vi "MiseEnFormeStreamMesuresValise.vi"(4 "Error In":errorcluster caption="Entrée d'erreur", 6 "MesuresBrutesValise":dbl[](array[numeric])=[1.0, 1.0, 1.0, 1.0, 1.0, 1.0, 1.0, 1.0, 1.0, 1.0, 1.0, 1.0, 1.0, 1.0, 1.0, 1.0, 1.0, 1.0, 1.0, 1.0, 1.0, 1.0, 1.0, 1.0], 7 "ConfigTotale":T1={"VoltageChannels"={"ChannelNames"=["capteur1", "capteur2"], "Sensitivity(Unit/V)"=[1.0, 1.0], "AutoZero"=[FALSE, FALSE], "ChannelUnits"=["V", "V"], "Offsets(Units)"=[0.0, 0.0], "Graph Num"=[]}, "WheastoneBridgeChannels"={"ChannelNames"=["capteur1", "capteur2"], "Sensitivity(Unit/V)"=[1.0, 1.0], "AutoZero"=[FALSE, FALSE], "ChannelUnits"=["V", "V"], "Offsets(Units)"=[0.0, 0.0], "Graph Num"=[]}, "Configuration"={"AcqSamplingRate(Hz)"=1000, "AcqTime(s)"=10, "Trigger"=FALSE, "NbVoltageChannels"=2, "NbWBridgeChannels"=2, "Qualisys"=FALSE, "Hexapode"=FALSE, "FinalSamplingRate(Hz)"=100, "QualisysDataType"=enum."6DOF", "Nortek"=FALSE, "HBM"=FALSE}}) -> (0 "Error Out":errorcluster caption="Sortie d'erreur", 2 "VoltageChannels1(0to15)":dbl[](array[numeric])=[1.0, 1.0], 3 "WBridgeChannels":dbl[](array[numeric])=[1000.0, 1000.0])   [LabVIEW 2017]
uses:
  DefDeType/ConfigTotale.ctl
  DefDeType/VoltageChannels.ctl
  DefDeType/WBridgeChannels.ctl
  DefDeType/Configuration.ctl
panel:
  out "size(s)":i32
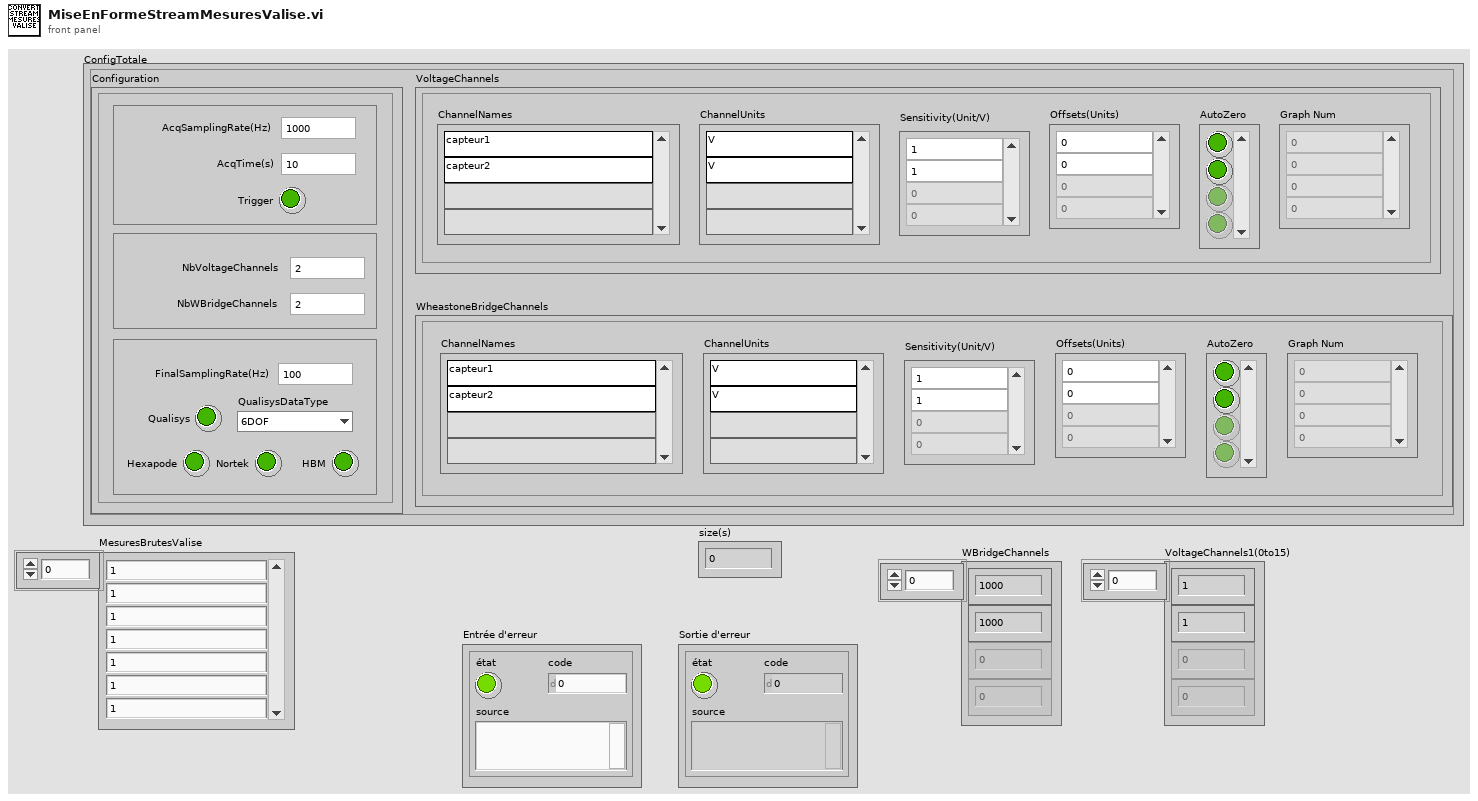
[diagram p1: front panel]
types:
  T1 = typedef "ConfigTotale.ctl" = cluster{"VoltageChannels":T2, "WheastoneBridgeChannels":T3, "Configuration":T4}
  T2 = typedef "VoltageChannels.ctl" = cluster{"ChannelNames":string[], "Sensitivity(Unit/V)":dbl[], "AutoZero":bool[], "ChannelUnits":string[], "Offsets(Units)":dbl[], "Graph Num":u8[]}
  T3 = typedef "WBridgeChannels.ctl" = cluster{"ChannelNames":string[], "Sensitivity(Unit/V)":dbl[], "AutoZero":bool[], "ChannelUnits":string[], "Offsets(Units)":dbl[], "Graph Num":u8[]}
  T4 = typedef "Configuration.ctl" = cluster{"AcqSamplingRate(Hz)":u32, "AcqTime(s)":u32, "Trigger":bool, "NbVoltageChannels":u32, "NbWBridgeChannels":u32, "Qualisys":bool, "Hexapode":bool, "FinalSamplingRate(Hz)":u32, "QualisysDataType":enum16{"6DOF", "3DTracking", "6DOF + 3D"}, "Nortek":bool, "HBM":bool}
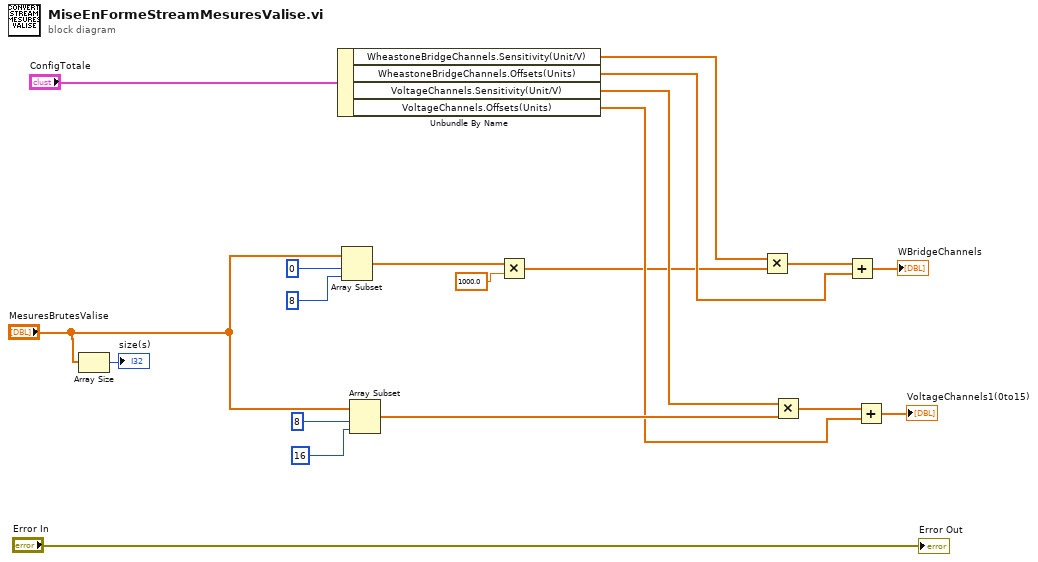
[diagram p0: block diagram]
diagram:
  n1 = Array Size(array="MesuresBrutesValise") -> (size(s)=→"size(s)":i32)
  n2 = Unbundle By Name("ConfigTotale") -> ("WheastoneBridgeChannels.Sensitivity(Unit/V)"=w13:dbl[], "WheastoneBridgeChannels.Offsets(Units)"=w12:dbl[], "VoltageChannels.Sensitivity(Unit/V)"=w15:dbl[], "VoltageChannels.Offsets(Units)"=w11:dbl[])
  n3 = Array Subset(array="MesuresBrutesValise", index=0 ("indice"), length=8 ("longueur")) -> (w4:dbl[])
  n4 = Array Subset(array="MesuresBrutesValise", index=8 ("indice"), length=16 ("longueur")) -> (w16:dbl[])
  n5 = Multiply(x=w4, y=1000.0) -> (x*y=w5:dbl[])
  n6 = Multiply(x=w13, y=w5) -> (x*y=w14:dbl[])
  n7 = Multiply(x=w15, y=w16) -> (x*y=w10:dbl[])
  n8 = Add(x=w14, y=w12) -> (x+y=→"WBridgeChannels":dbl[])
  n9 = Add(x=w10, y=w11) -> (x+y=→"VoltageChannels1(0to15)":dbl[])
  "Error Out" <- "Error In"
